vi "PathPlanner_Cmd_FindFollowRamsetePathSimpleExecute.vi"(5 "PathPlanner_Cmd_FollowRamConfig":T10={"ControlPastEnd_Sec"=3.0, "ReplanningConfig"={"enableInitialReplanning"=TRUE, "enableDynamicReplanning"=FALSE, "dynamicReplanningTotalErrorThreshold"=1.0, "dynamicReplanningErrorSpikeThreshold"=0.25}, "Trigger Events"=TRUE, "RAMSETE_EXE_TUNING SI"={"B"=2.0, "Zeta"=0.7, "X Tolerance M"=2.0, "Y Tolerance M"=0.7, "Heading Tolerance RAD"=0.7, "Track Width M"=2.0, "Max Speed M/S"=2.0}} {"RAMSETE_EXE_TUNING SI"."Max Speed M/S" format="%13.4f"; "RAMSETE_EXE_TUNING SI"."Track Width M" format="%13.4f"; "RAMSETE_EXE_TUNING SI"."Heading Tolerance RAD" format="%13.4f"; "RAMSETE_EXE_TUNING SI"."Y Tolerance M" format="%13.4f"; "RAMSETE_EXE_TUNING SI"."X Tolerance M" format="%13.4f"; "RAMSETE_EXE_TUNING SI"."Zeta" format="%13.4f"; "RAMSETE_EXE_TUNING SI"."B" format="%13.4f"}, 6 "PassthroughTime_SEC":dbl=-1.0, 7 "PathPlanner_Cmd_FindConfig":T1={"Goal Position"={"X"=0.0, "Y"=0.0}, "GoalEndState"={"VelocityMPS"=0.0, "Rotation"={"VALUE"=0.0, "COS"=1.0, "SIN"=0.0}}, "PathPlannerPathConstraints"={"MaxVelocityMps;"=0.0, "MaxAccelerationMpsSq;"=0.0, "MaxAngularVelRadPsEc;"=0.0, "MaxAngularAccRadPSecSq"=0.0, "Exists"=FALSE, "Unlimited"=FALSE, "NominalVoltageVolts"=12.0}, "Rotation Delay Distance M"=0.0} {"GoalEndState"."Rotation"."SIN" format="%13.4f"; "GoalEndState"."Rotation"."COS" format="%13.4f"; "GoalEndState"."Rotation"."VALUE" format="%13.4f"; "Goal Position"."Y" step=0.25 format="%14.3f"; "Goal Position"."X" format="%14.3f"}, 8 "Enabled":bool=TRUE, 9 "Reset":bool, 10 "CurrentChassisSpeeds":T9 {"vOmega" format="%10.3f"; "vY" format="%10.3f"; "vX" format="%10.3f"}, 11 "Current Pose SI":T8={"TRANSLATION"={"X"=0.0, "Y"=0.0}, "ROTATION"={"VALUE"=0.0, "COS"=1.0, "SIN"=0.0}} {"ROTATION"."SIN" format="%13.4f"; "ROTATION"."COS" format="%13.4f"; "ROTATION"."VALUE" format="%13.4f"; "TRANSLATION"."Y" format="%14.3f"; "TRANSLATION"."X" format="%14.3f"}) -> (0 "Position Error M":dbl, 1 "Complete":bool, 2 "At Reference":bool, 3 "Left Right Speed Dmds":T6, 4 "outRAMSETE":T7={"B"=2.0, "Zeta"=0.7, "poseTolerance"={"TRANSLATION"={"X"=0.0, "Y"=0.0}, "ROTATION"={"VALUE"=0.0, "COS"=1.0, "SIN"=0.0}}, "poseError"={"TRANSLATION"={"X"=0.0, "Y"=0.0}, "ROTATION"={"VALUE"=0.0, "COS"=1.0, "SIN"=0.0}}, "Enabled"=TRUE} {"poseError"."ROTATION"."SIN" format="%13.4f"; "poseError"."ROTATION"."COS" format="%13.4f"; "poseError"."ROTATION"."VALUE" format="%13.4f"; "poseError"."TRANSLATION"."Y" format="%14.3f"; "poseError"."TRANSLATION"."X" format="%14.3f"; "poseTolerance"."ROTATION"."SIN" format="%13.4f"; "poseTolerance"."ROTATION"."COS" format="%13.4f"; "poseTolerance"."ROTATION"."VALUE" format="%13.4f"; "poseTolerance"."TRANSLATION"."Y" format="%14.3f"; "poseTolerance"."TRANSLATION"."X" format="%14.3f"; "Zeta" format="%12.3f"; "B" format="%12.3f"})   [LabVIEW 2019, in "PathPlanner24.lvlib"]
doc: "DOCUMENTATION IS NOT COMPLETE.\n\nFind and follow a path for differential drive robots using Ramsete controller.\n \n\nInputs:\n - CurrentPoseSi - pose2d - The current pose calculated by odometry or pose estimation. The pose can be absolute or relative depending on what type of trajectory is being followed.\n - Reset - boolean - When TRUE the holonomic drive controller is reset. This should be set to TRUE for the first execution of a trajectory.\n - Enabled - boolean - When TRUE, closed loop control is enabled. (Optional. Default: TRUE)\n\nOutputs:\n - AtReference - boolean - TRUE if the robots position is within the defined tolerance.\n - PositionError - pose2d - Position error in SI units. How far the robot is away from the desired trajectory position."
uses:
  PathPlanner24.lvlib
  <vilib>/Rock Robotics/WPI/ThirdParty/JAS_Junk/TrajLib/TypeDef/POSE2D.ctl
  <vilib>/Rock Robotics/WPI/ThirdParty/JAS_Junk/TrajLib/TypeDef/TRANSLATION2D.ctl
  <vilib>/Rock Robotics/WPI/ThirdParty/JAS_Junk/TrajLib/TypeDef/ROTATION2D.ctl
  TypeDef/PathPlannerCmdFollowRamConfig.ctl
  TypeDef/PathPlannerReplanningConfig.ctl
  <vilib>/Rock Robotics/WPI/ThirdParty/JAS_Junk/TrajLib/TypeDef/RAMSETE_EXE_TUNING.ctl
  <vilib>/Rock Robotics/WPI/ThirdParty/JAS_Junk/TrajLib/TypeDef/CHASSIS_SPEEDS.ctl
  <vilib>/Rock Robotics/WPI/ThirdParty/JAS_Junk/TrajLib/TypeDef/RAMSETE.ctl
  TypeDef/PathPlannerCmdFindConfig.ctl
  TypeDef/PathPlannerGoalEndState.ctl
  TypeDef/PathPlannerPathConstraints.ctl
  <vilib>/Rock Robotics/WPI/ThirdParty/JAS_Junk/TrajLib/Util_CalcDist.vi
  <vilib>/Rock Robotics/WPI/ThirdParty/JAS_Junk/TrajLib/Trajectory_Library.lvlib
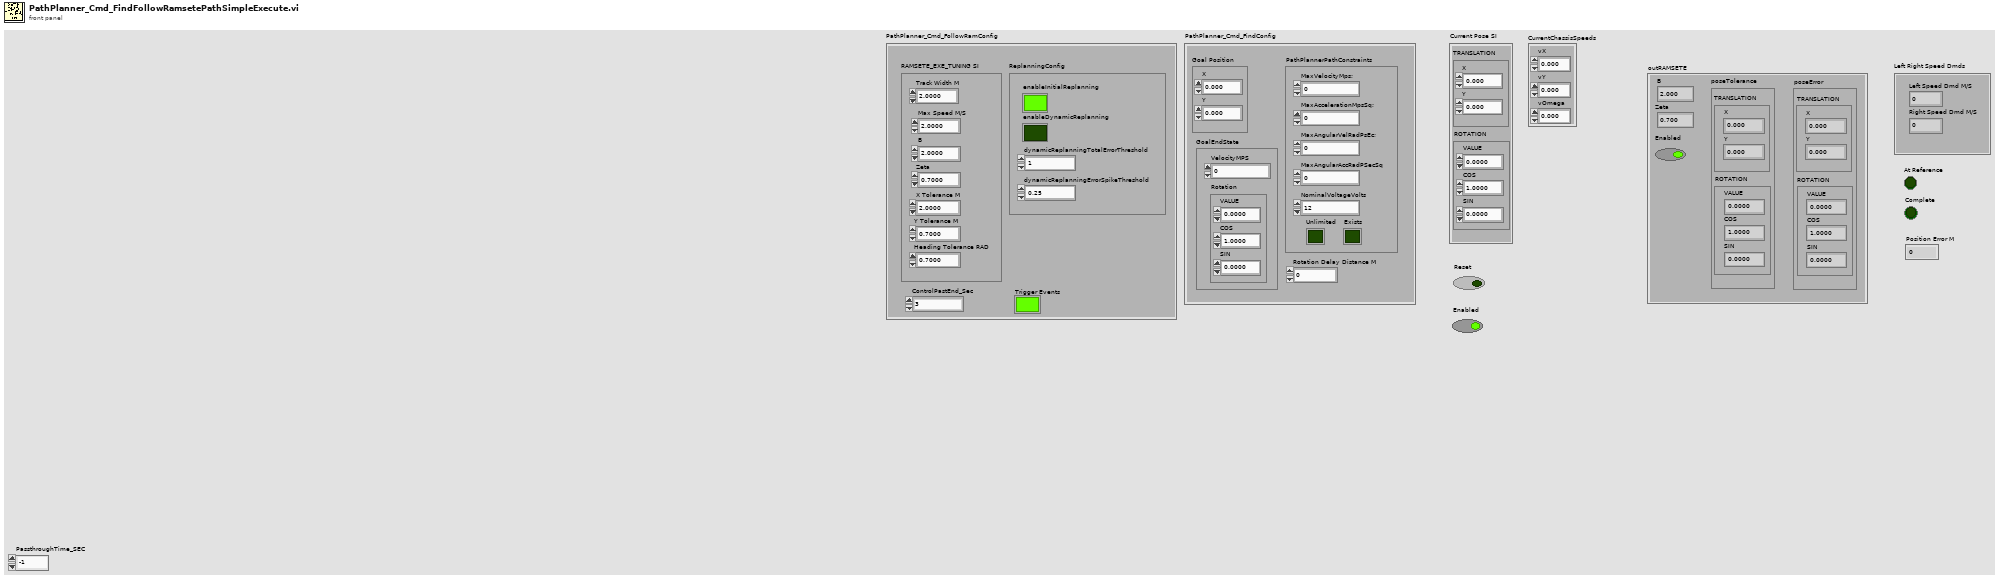
[diagram p1: front panel]
types:
  T1 = typedef "PathPlanner24.lvlib/PathPlannerCmdFindConfig.ctl" = cluster{"Goal Position":T2, "GoalEndState":T3, "PathPlannerPathConstraints":T5, "Rotation Delay Distance M":dbl}
  T2 = typedef "Trajectory_Library.lvlib/TRANSLATION2D.ctl" = cluster{"X":dbl, "Y":dbl}
  T3 = typedef "PathPlanner24.lvlib/PathPlannerGoalEndState.ctl" = cluster{"VelocityMPS":dbl, "Rotation":T4}
  T4 = typedef "Trajectory_Library.lvlib/ROTATION2D.ctl" = cluster{"VALUE":dbl, "COS":dbl, "SIN":dbl}
  T5 = typedef "PathPlanner24.lvlib/PathPlannerPathConstraints.ctl" = cluster{"MaxVelocityMps;":dbl, "MaxAccelerationMpsSq;":dbl, "MaxAngularVelRadPsEc;":dbl, "MaxAngularAccRadPSecSq":dbl, "Exists":bool, "Unlimited":bool, "NominalVoltageVolts":dbl}
  T6 = cluster{"Left Speed Dmd M/S":dbl, "Right Speed Dmd M/S":dbl}
  T7 = typedef "Trajectory_Library.lvlib/RAMSETE.ctl" = cluster{"B":dbl, "Zeta":dbl, "poseTolerance":T8, "poseError":T8, "Enabled":bool}
  T8 = typedef "Trajectory_Library.lvlib/POSE2D.ctl" = cluster{"TRANSLATION":T2, "ROTATION":T4}
  T9 = typedef "Trajectory_Library.lvlib/CHASSIS_SPEEDS.ctl" = cluster{"vX":dbl, "vY":dbl, "vOmega":dbl}
  T10 = typedef "PathPlanner24.lvlib/PathPlannerCmdFollowRamConfig.ctl" = cluster{"ControlPastEnd_Sec":dbl, "ReplanningConfig":T11, "Trigger Events":bool, "RAMSETE_EXE_TUNING SI":T12}
  T11 = typedef "PathPlanner24.lvlib/PathPlannerReplanningConfig.ctl" = cluster{"enableInitialReplanning":bool, "enableDynamicReplanning":bool, "dynamicReplanningTotalErrorThreshold":dbl, "dynamicReplanningErrorSpikeThreshold":dbl}
  T12 = typedef "Trajectory_Library.lvlib/RAMSETE_EXE_TUNING.ctl" = cluster{"B":dbl, "Zeta":dbl, "X Tolerance M":dbl, "Y Tolerance M":dbl, "Heading Tolerance RAD":dbl, "Track Width M":dbl, "Max Speed M/S":dbl}
  T13 = typedef "PathPlanner24.lvlib/PathPlannerPath.ctl" = cluster{"Reversed":bool, "RotationTargets":T14[], "ConstraintZones":T15[], "EventMarkers":T16[], "GlobalConstraints":T5, "GoalEndState":T3, "AllPoints":T19[], "Name":string, "Waypoints":T20[], "PointTowardsZones":T21[], "IdealStartingState":T22, "IsChoreoPath":bool, "PreventFlipping":bool}
  T14 = typedef "PathPlanner24.lvlib/PathPlannerRotationTarget.ctl" = cluster{"position":dbl, "rotation":T4, "Exists":bool}
  T15 = typedef "PathPlanner24.lvlib/PathPlannerConstraintsZone.ctl" = cluster{"minPosition":dbl, "maxPosition":dbl, "Constraints":T5, "Present":bool}
  T16 = typedef "PathPlanner24.lvlib/PathPlannerEventMarker.ctl" = cluster{"Position":dbl, "Command":T17, "TriggerName":string, "EndPosition":dbl}
  T17 = typedef "PathPlanner24.lvlib/PathPlannerCommandUtil.ctl" = cluster{"waitTime":dbl, "name":string, "pathName":string, "commands":cluster{"type":T18, "waitTime":dbl, "name":string, "pathName":string}[], "type":T18}
  T18 = typedef "PathPlanner24.lvlib/PathPlanner_CommandUtilType_ENUM.ctl" = enum16{"Unknown", "Wait", "Named", "Path", "Sequential", "Parallel", "Race", "Deadline"}
  T19 = typedef "PathPlanner24.lvlib/PathPlannerPathPoint.ctl" = cluster{"Position":T2, "DistAlongPath":dbl, "MaxV":dbl, "Constraints":T5, "RotationTarget":T14, "WaypointRelativePos":dbl}
  T20 = typedef "PathPlanner24.lvlib/PathPlannerWaypoint.ctl" = cluster{"prevControl":T2, "anchor":T2, "nextControl":T2, "PrevExists":bool, "NextExists":bool}
  T21 = typedef "PathPlanner24.lvlib/PathPlannerPointTowardsZone.ctl" = cluster{"RotationOffset":T4, "Name":string, "TargetPosition":T2, "MinPosition":dbl, "MaxPosition":dbl}
  T22 = typedef "PathPlanner24.lvlib/PathPlannerIdealStartingState.ctl" = cluster{"VelocityMPS":dbl, "Rotation":T4}
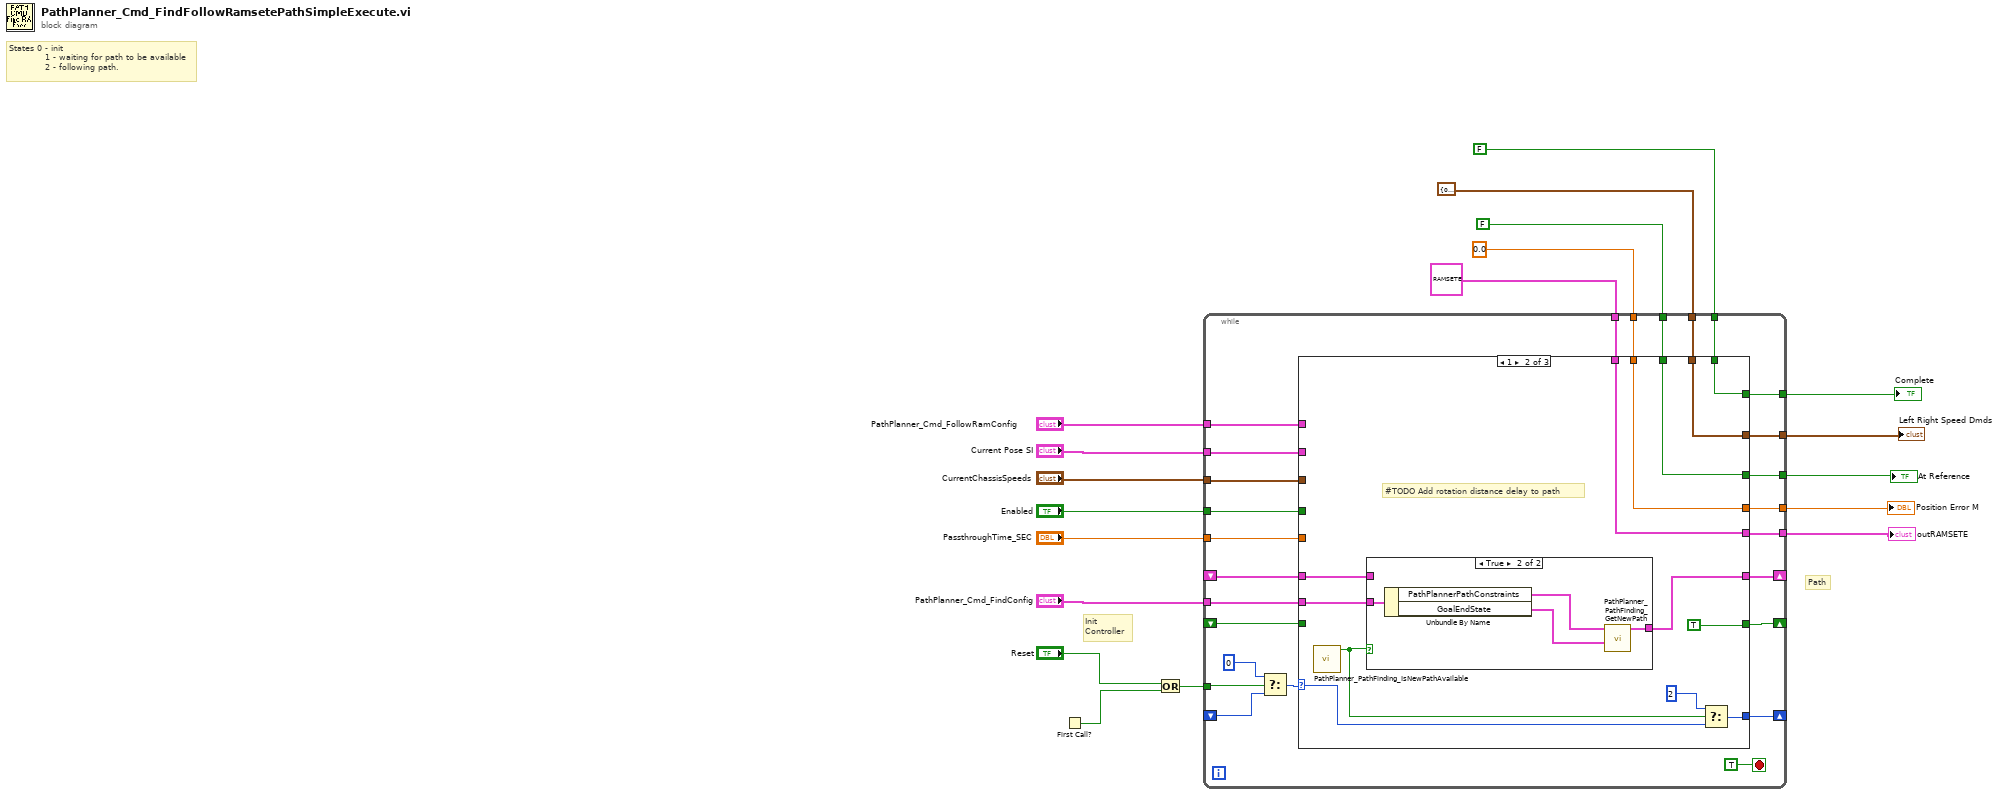
[diagram p0: block diagram]
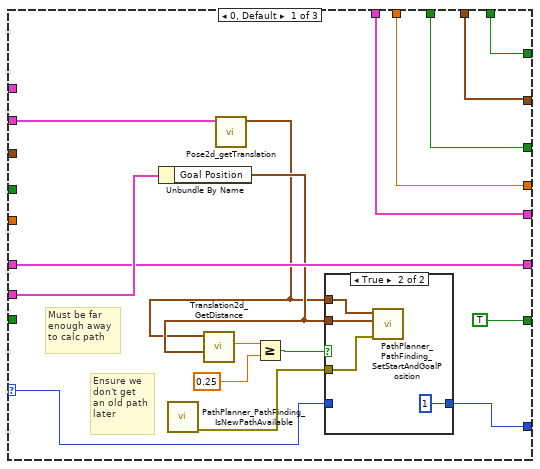
[diagram p2: hidden frame]
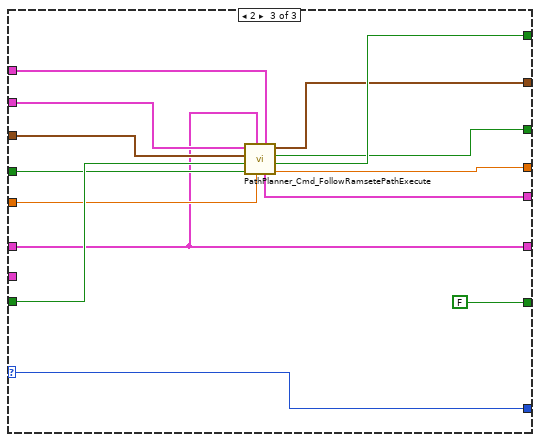
[diagram p5: hidden frame]
diagram:
  # "Init\nController"
  # "Path"
  # "States 0 - init \n            1 - waiting for path to be available\n            2 - following path."
  n1 = First Call?() -> (First Call?: T/F=w19:bool)
  n2 = Or(x="Reset", y=w19) -> (x .or. y?=w18:bool)
  n3 = while {
    tunnel: "PathPlanner_Cmd_FollowRamConfig" -> [w29]
    tunnel: "Current Pose SI" -> [w37]
    tunnel: "Enabled" -> [w44]
    tunnel: [w40] -> w13
    tunnel: "CurrentChassisSpeeds" -> [w43]
    shift-right: [w38] -> _
    shift-left: _ -> [w41]
    tunnel: "PassthroughTime_SEC" -> [w42]
    tunnel: [w39] -> w14
    tunnel: w18 -> [w36]
    shift-right: [w32] -> _
    shift-left: _ -> [w33]
    tunnel: "PathPlanner_Cmd_FindConfig" -> [w31]
    shift-right: [w30] -> _
    shift-left: _ -> [w28]
    tunnel: [w27] -> w12
    tunnel: T7 {"B"=2.0, "Zeta"=0.7, "poseTolerance"={"TRANSLATION"={"X"=0.0, "Y"=0.0}, "ROTATION"={"VALUE"=0.0, "COS"=1.0, "SIN"=0.0}}, "poseError"={"TRANSLATION"={"X"=0.0, "Y"=0.0}, "ROTATION"={"VALUE"=0.0, "COS"=1.0, "SIN"=0.0}}, "Enabled"=TRUE} ("outRAMSETE") -> [w26]
    tunnel: FALSE ("Complete") -> [w25]
    tunnel: T6 {"Left Speed Dmd M/S"=0.0, "Right Speed Dmd M/S"=0.0} ("Left Right Speed Dmds") -> [w24]
    tunnel: FALSE ("At Reference") -> [w23]
    tunnel: 0.0 ("Position Error M") -> [w22]
    tunnel: [w21] -> w10
    tunnel: [w20] -> w2
    stop <- TRUE stop-if-true
    n4 = Select(t=0, s=w36, f=w33) -> (s? t:f=w34:i32)
    n5 = case shown="1" w34 {
      selector: w34 -> [w48 w70 w88]
      tunnel: w44 -> [_ _ w92]
      tunnel: [w60 w74 w96] -> w27
      tunnel: w43 -> [_ _ w94]
      tunnel: w42 -> [_ _ w91]
      tunnel: w41 -> [w58 w76 w89]
      tunnel: [w59 w73 w97] -> w40
      tunnel: [w56 w72 w98] -> w39
      tunnel: [w58 w77 w89] -> w38
      tunnel: w37 -> [w57 _ w95]
      tunnel: [w49 w71 w88] -> w32
      tunnel: w31 -> [w62 w78 _]
      tunnel: [TRUE TRUE FALSE] -> w30
      tunnel: w29 -> [_ _ w90]
      tunnel: w28 -> [_ _ w93]
      tunnel: w22 -> [w60 w74 _]
      tunnel: w23 -> [w59 w73 _]
      tunnel: w24 -> [w47 w69 _]
      tunnel: w25 -> [w56 w72 _]
      tunnel: w26 -> [w46 w68 _]
      tunnel: [w46 w68 w87] -> w21
      tunnel: [w47 w69 w86] -> w20
      frame 0, Default {
        # "Must be far\nenough away\nto calc path"
        # "Ensure we\ndon't get\nan old path\nlater"
        n6 = Unbundle By Name(w62) -> ("Goal Position"=w52:T2)
        n7 = call "PathPlanner_PathFinding_IsNewPathAvailable.vi"() -> ("error out"=w51:errorcluster)  [unwired: 10 in, 1 out]
        n8 = call <vilib>:"Pose2d_getTranslation.vi"("in POSE"=w57) -> ("outTRANSLATION"=w50:T2)  [unwired: 10 in]
        n9 = call <vilib>:"Translation2d_GetDistance.vi"("other Translation"=w52, "In Translation"=w50) -> ("Distance"=w55:dbl)  [unwired: 9 in]
        n10 = Greater Or Equal?(x=w55, y=0.25) -> (x >= y?=w53:bool)
        n11 = case shown="True" w53 {
          tunnel: w52 -> [_ w67]
          tunnel: w51 -> [_ w66]
          tunnel: w50 -> [_ w65]
          tunnel: [w63 1] -> w49
          tunnel: w48 -> [w63 _]
          frame False {
          }
          frame True {
            n12 = call "PathPlanner_PathFinding_SetStartAndGoalPosition.vi"("error in (no error)"=w66, "GoalPosition"=w67, "StartPosition"=w65) -> ()  [unwired: 8 in, 1 out]
          }
        }
      }
      frame 1 {
        # "#TODO Add rotation distance delay to path"
        n13 = call "PathPlanner_PathFinding_IsNewPathAvailable.vi"() -> ("New Path Available"=w79:bool)  [unwired: 10 in, 1 out]
        n14 = case shown="True" w79 {
          tunnel: w78 -> [_ w85]
          tunnel: [w81 w83] -> w77
          tunnel: w76 -> [w81 _]
          frame False {
          }
          frame True {
            n15 = Unbundle By Name(w85) -> ("PathPlannerPathConstraints"=w82:T5, "GoalEndState"=w84:T3)
            n16 = call "PathPlanner_PathFinding_GetNewPath.vi"("GoalEndState"=w84, "PathPlannerPathConstraints"=w82) -> ("PathPlannerPath"=w83:T13)  [unwired: 8 in, 1 out]
          }
        }
        n17 = Select(t=2, s=w79, f=w70) -> (s? t:f=w71:i32)
      }
      frame 2 {
        n18 = call "PathPlanner_Cmd_FollowRamsetePathExecute.vi"("PathPlanner_Cmd_FollowRamConfig"=w90, "PassthroughTime_SEC"=w91, "PathPlannerPath"=w89, "Enabled"=w92, "Reset"=w93, "CurrentChassisSpeeds"=w94, "Current Pose SI"=w95) -> ("Position Error M"=w96:dbl, "Complete"=w98:bool, "At Reference"=w97:bool, "Left Right Speed Dmds"=w86:T6, "outRAMSETE"=w87:T7)
      }
    }
  }
  "At Reference" <- w13
  "Position Error M" <- w12
  "Complete" <- w14
  "outRAMSETE" <- w10
  "Left Right Speed Dmds" <- w2
